vi "公式节点.vi"() -> ()   [LabVIEW 2017]
panel:
  out "XY图 2":cluster{i32, "y2":dbl}[](graph)
  out "XY图":cluster{i32, "y1":dbl}[](graph)
  out "循环次数":i32
  out "y2":dbl
  out "y1":dbl
  in  "b":dbl
  in  "a":dbl
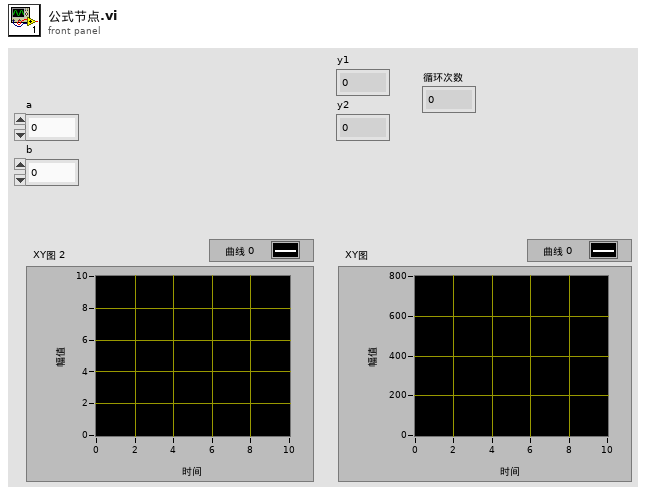
[diagram p1: front panel]
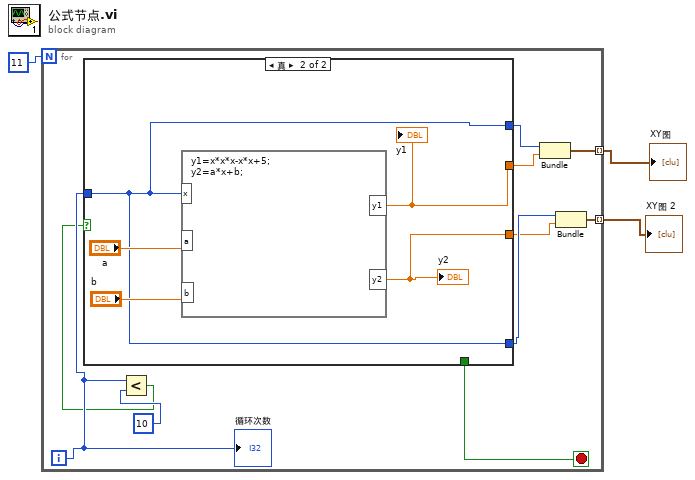
[diagram p0: block diagram]
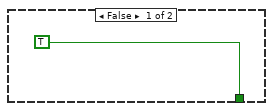
[diagram p2: hidden frame]
diagram:
  n1 = for {
    N: 11 -> [_]
    tunnel: [w6] -> w2 mode=indexing
    tunnel: [w5] -> w1 mode=indexing
    i -> [w12]
    stop <- w4 stop-if-true
    n2 = Less?(x=w12, y=10) -> (x < y?=w11:bool)
    n3 = case shown="真" w11 {
      tunnel: w12 -> [_ w16]
      tunnel: [_ w16] -> w10
      tunnel: [_ w17] -> w9
      tunnel: [_ w16] -> w8
      tunnel: [_ w15] -> w7
      tunnel: [TRUE _] -> w4
      frame False {
      }
      frame True {
        n4 = formula code="y1=x*x*x-x*x+5;\ny2=a*x+b;"("a"="a", "b"="b", "x"=w16) -> ("y1"=w17:dbl, "y2"=w15:dbl)
        "y1" <- w17
        "y2" <- w15
      }
    }
    n5 = Bundle(w10, "y1"=w9) -> (w6:cluster{i32, "y1":dbl})  [unwired: 1 in]
    n6 = Bundle(w8, "y2"=w7) -> (w5:cluster{i32, "y2":dbl})  [unwired: 1 in]
    "循环次数" <- w12
  }
  "XY图" <- w2
  "XY图 2" <- w1
